vi "Deform_Mirror_ae.vi"(0 "Refnum In":refnum<k7>, 1 "Enum":enum16{"WRITE", "READ"}(ring), 5 "IDs In":i32[](array[numeric]), 7 "Flat Files In":dbl[][](array[numeric]), 9 "Multi Map Data In":i32[](array[numeric]), 11 "Mode Matrix In":T1) -> (4 "Refnum Out":refnum<k7>, 6 "IDs Out":i32[](array[numeric]), 8 "Flat Files Out":dbl[][](array[numeric]), 10 "Multi Map Data Out":i32[](array[numeric]), 15 "Mode Matrix Out":T1)   [LabVIEW 2015]
uses:
  <vilib>/Analysis/Matrix/Datatypes/RealMatrix.ctl
  <vilib>/Analysis/Matrix/NI_Matrix.lvlib
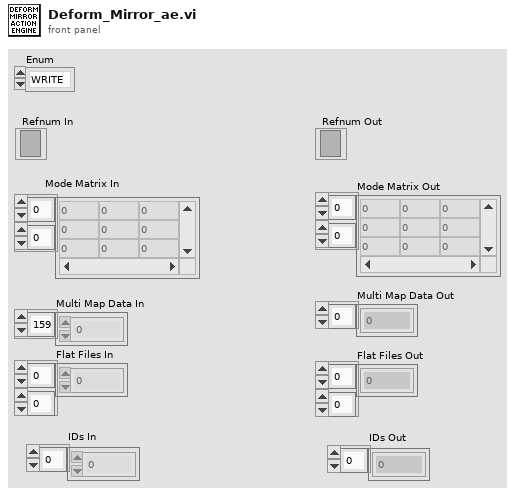
[diagram p1: front panel]
types:
  T1 = typedef "NI_Matrix.lvlib/RealMatrix.ctl" = dbl[][]
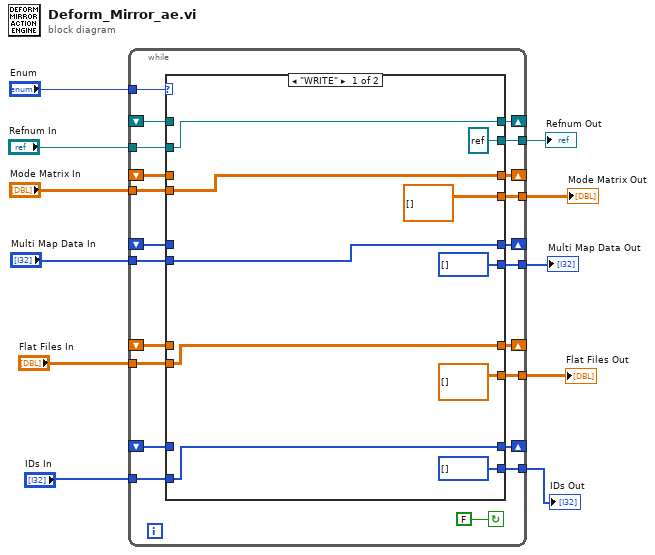
[diagram p0: block diagram]
diagram:
  n1 = while {
    tunnel: "Enum" -> [w32]
    shift-right: [w20] -> _
    shift-left: _ -> [w31]
    tunnel: "Flat Files In" -> [w30]
    shift-right: [w18] -> _
    shift-left: _ -> [w29]
    shift-right: [w28] -> _
    shift-left: _ -> [w25]
    tunnel: "Mode Matrix In" -> [w27]
    tunnel: [w26] -> w9
    shift-right: [w24] -> _
    shift-left: _ -> [w22]
    tunnel: "Multi Map Data In" -> [w23]
    tunnel: [w21] -> w7
    tunnel: [w19] -> w5
    tunnel: "IDs In" -> [w17]
    tunnel: [w16] -> w1
    shift-right: [w15] -> _
    shift-left: _ -> [w13]
    tunnel: "Refnum In" -> [w14]
    tunnel: [w12] -> w3
    stop <- FALSE continue-if-true
    n2 = case shown="\"WRITE\"" w32 {
      tunnel: w31 -> [_ w46]
      tunnel: w30 -> [w39 _]
      tunnel: w29 -> [_ w45]
      tunnel: [w43 w48] -> w28
      tunnel: w27 -> [w43 _]
      tunnel: [T1 [] ("Mode Matrix IN") w48] -> w26
      tunnel: w25 -> [_ w48]
      tunnel: [w41 w47] -> w24
      tunnel: w23 -> [w41 _]
      tunnel: w22 -> [_ w47]
      tunnel: [i32[] [] ("Multi Map Data In") w47] -> w21
      tunnel: [w39 w46] -> w20
      tunnel: [dbl[][] [] ("Flat Files In") w46] -> w19
      tunnel: [w38 w45] -> w18
      tunnel: w17 -> [w38 _]
      tunnel: [i32[] [] ("IDs In") w45] -> w16
      tunnel: [w37 w44] -> w15
      tunnel: w14 -> [w37 _]
      tunnel: w13 -> [_ w44]
      tunnel: [refnum<k7> refnum ("Refnum In") w44] -> w12
      frame "WRITE" {
      }
      frame "READ" {
      }
    }
  }
  "Flat Files Out" <- w5
  "Mode Matrix Out" <- w9
  "Multi Map Data Out" <- w7
  "Refnum Out" <- w3
  "IDs Out" <- w1
